vi "NML data acq file header lines.vi"(11 "all rows":dbl[][](array[numeric])=[[0.0, 0.0, 0.0, 0.0, 0.0, 0.0], [0.0, 0.0, 0.0, 0.0, 0.0, 0.0], [0.0, 1.0, 1.0, 1.0, 1.0, 1.0], [0.0, 1.0, 0.1, 0.11, 0.212, 0.55], [0.0, 0.0, 0.0, 0.0, 0.0, 0.0], [0.0, 0.0, 0.0, 0.0, 0.0, 0.0], [0.0, 0.0, 0.0, 0.0, 0.0, 0.0]]) -> (1 "real data?":dbl[][](array[numeric]), 2 "number of rows":i32, 3 "first good row":i32)   [LabVIEW 2019]
panel:
  in  "zero column check":bool
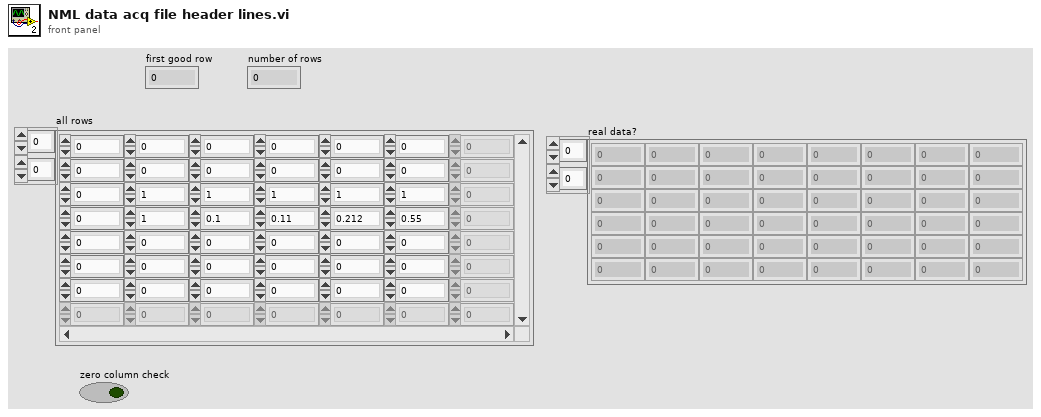
[diagram p1: front panel]
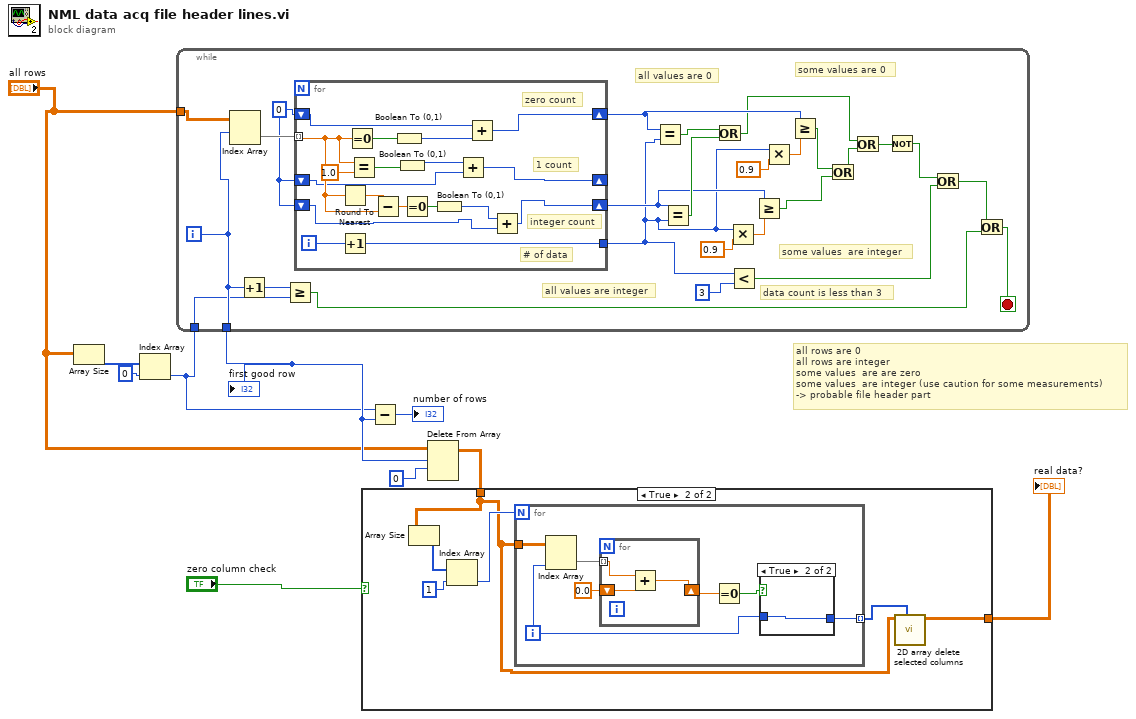
[diagram p0: block diagram]
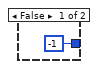
[diagram p3: hidden frame]
diagram:
  # "all rows are 0\nall rows are integer\nsome values  are are zero\nsome values  are integer (use caution for some measurements)\n-> probable file header part"
  n1 = Array Size(array="all rows") -> (size(s)=w10:i32[])
  n2 = Index Array(array=w10, index=0) -> (element=w5:i32)
  n3 = while {
    tunnel: "all rows" -> [w36]
    tunnel: [w16] -> w6
    tunnel: w5 -> [w15]
    i -> [w16]
    stop <- w11 stop-if-true
    w34 = i16 0
    # "data count is less than 3"
    # "some values are 0"
    # "some values  are integer"
    # "all values are integer"
    # "all values are 0"
    n4 = Index Array(array=w36, index (row)=w16) -> (element=w35:dbl[])  [unwired: 1 in]
    n5 = Increment(x=w16) -> (x+1=w14:i32)
    n6 = Greater Or Equal?(x=w14, y=w15) -> (x >= y?=w12:bool)
    n7 = for {
      tunnel: w35 -> [w53] mode=indexing
      shift-right: [w45] -> w27
      shift-left: w34 -> [w46]
      shift-right: [w39] -> _
      shift-left: w34 -> [w43]
      shift-right: [w40] -> w32
      shift-left: w34 -> [w41]
      tunnel: [w37] -> w21
      i -> [w38]
      # "# of data"
      # "integer count"
      # "1 count"
      # "zero count"
      n8 = Round To Nearest(number=w53) -> (nearest integer value=w54:dbl)
      n9 = Increment(x=w38) -> (x+1=w37:i32)
      n10 = Equal To 0?(x=w53) -> (x = 0?=w50:bool)
      n11 = Equal?(x=w53, y=1.0) -> (x = y?=w49:bool)
      n12 = Subtract(x=w54, y=w53) -> (x-y=w52:dbl)
      n13 = Boolean To (0,1)(Boolean=w50) -> (0, 1=w47:i16)
      n14 = Boolean To (0,1)(Boolean=w49) -> (0, 1=w44:i16)
      n15 = Equal To 0?(x=w52) -> (x = 0?=w48:bool)
      n16 = Boolean To (0,1)(Boolean=w48) -> (0, 1=w42:i16)
      n17 = Add(x=w44, y=w43) -> (x+y=w39:i16)
      n18 = Add(x=w46, y=w47) -> (x+y=w45:i16)
      n19 = Add(x=w42, y=w41) -> (x+y=w40:i16)
    }
    n20 = Equal?(x=w27, y=w21) -> (x = y?=w17:bool)
    n21 = Equal?(x=w32, y=w21) -> (x = y?=w33:bool)
    n22 = Or(x=w17, y=w33) -> (x .or. y?=w23:bool)
    n23 = Multiply(x=w21, y=0.9) -> (x*y=w30:dbl)
    n24 = Less?(x=w21, y=3) -> (x < y?=w18:bool)
    n25 = Greater Or Equal?(x=w32, y=w30) -> (x >= y?=w25:bool)
    n26 = Multiply(x=w21, y=0.9) -> (x*y=w28:dbl)
    n27 = Greater Or Equal?(x=w27, y=w28) -> (x >= y?=w26:bool)
    n28 = Or(x=w26, y=w25) -> (x .or. y?=w24:bool)
    n29 = Or(x=w23, y=w24) -> (x .or. y?=w22:bool)
    n30 = Not(x=w22) -> (.not. x?=w19:bool)
    n31 = Or(x=w19, y=w18) -> (x .or. y?=w13:bool)
    n32 = Or(x=w13, y=w12) -> (x .or. y?=w11:bool)
  }
  "first good row" <- w6
  n33 = Subtract(x=w5, y=w6) -> (x-y=→"number of rows":i32)
  n34 = Delete From Array(array="all rows", length=w6, index (row)=0) -> (array with subset deleted=w3:dbl[][])  [unwired: 1 in, 1 out]
  n35 = case shown="True" "zero column check" {
    tunnel: w3 -> [w55 w57]
    tunnel: [w55 w56] -> w1
    frame False {
    }
    frame True {
      n36 = Array Size(array=w57) -> (size(s)=w61:i32[])
      n37 = Index Array(array=w61, index=1) -> (element=w59:i32)
      n38 = for {
        N: w59 -> [_]
        tunnel: w57 -> [w65]
        tunnel: [w63] -> w58 mode=indexing
        i -> [w62]
        n39 = Index Array(array=w65, index (col)=w62) -> (element=w66:dbl[])  [unwired: 1 in]
        n40 = for {
          tunnel: w66 -> [w73] mode=indexing
          shift-right: [w71] -> w68
          shift-left: 0.0 -> [w72]
          n41 = Add(x=w73, y=w72) -> (x+y=w71:dbl)
        }
        n42 = Equal To 0?(x=w68) -> (x = 0?=w64:bool)
        n43 = case shown="True" w64 {
          tunnel: [-1 w70] -> w63
          tunnel: w62 -> [_ w70]
          frame False {
          }
          frame True {
          }
        }
      }
      n44 = call "2D array delete selected columns.vi"("colums to be deleted"=w58, "input 2d array"=w57) -> ("output 2d array"=w56:dbl[][])  [unwired: 9 in]
    }
  }
  "real data?" <- w1
